vi "command_mapping.vi"(0 "Controls[]":refnum<vi>[](array[refnum]), 2 "cmd in":string, 3 "connection information":path) -> (8 "address out":i16, 9 "value out":T1)   [LabVIEW 2015]
uses:
  Control 1.ctl
  <vilib>/addons/database/Connection.llb/DB Tools Open Connec (Path).vi
  <vilib>/Utility/Data Type/NI_Data Type.lvlib
  <vilib>/addons/database/NI_Database_API.lvlib
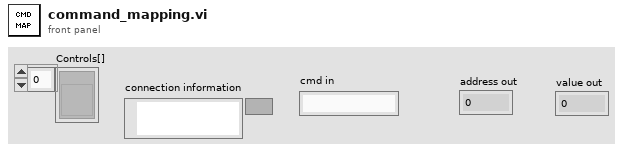
[diagram p1: front panel]
types:
  T1 = typedef "Control 1.ctl" = dbl
  T2 = typedef "NI_Data Type.lvlib/Data Type.ctl" = enum8{"Invalid Type", "Void", "I8", "I16", "I32", "I64", "U8", "U16", "U32", "U64", "Single Float", "Double Float", "Extended Float", "Single Complex", "Double Complex", "Extended Complex", "Enum U8", "Enum U16", "Enum U32", "Enum U64", "Single Float With Unit", "Double Float With Unit", "Extended Float With Unit", "Single Complex with Unit", "Double Complex with Unit", "Extended Complex with Unit", "Boolean", "String", "Path", "Picture", "Tag", "Array", "Cluster", "Variant", "LV Variant", "Waveform", "Timestamp", "Digital Waveform", "Digital Data", "ExpressData", "Refnum", "External Data", "VI", "Poly VI", "LabVIEW Class Instance", "Fixed Point"}
  T3 = typedef "NI_Database_API.lvlib/Conn ObjectReference.ctl" = refnum<k1>
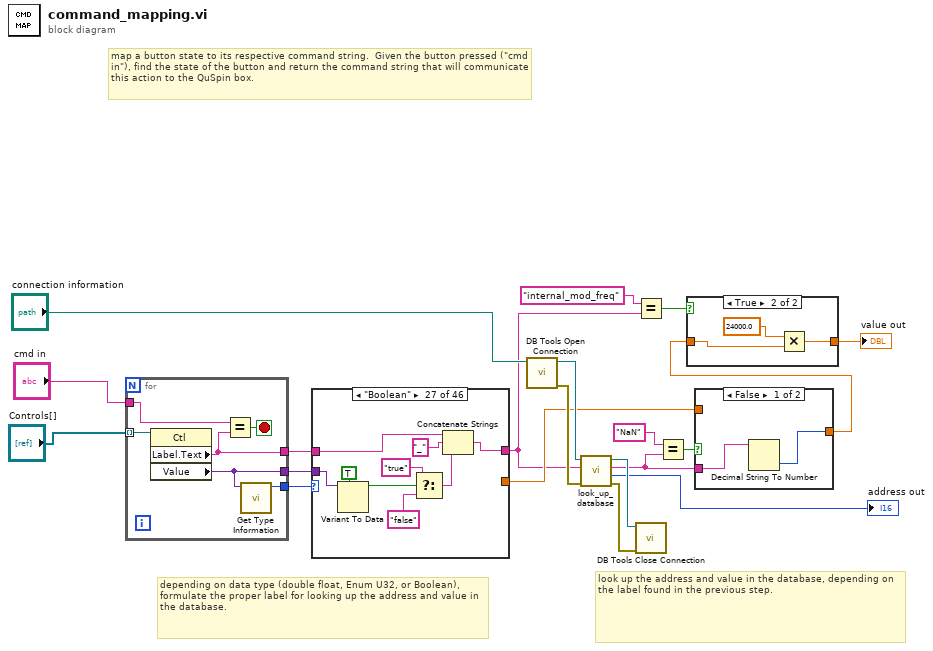
[diagram p0: block diagram]
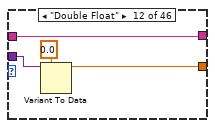
[diagram p15: hidden frame]
diagram:
  # "look up the address and value in the database, depending on the label found in the previous step."
  # "depending on data type (double float, Enum U32, or Boolean), formulate the proper label for looking up the address and value in the database."
  # "map a button state to its respective command string.  Given the button pressed (\"cmd in\"), find the state of the button and return the command string that will communicate this action to the QuSpin box."
  n1 = for {
    tunnel: "Controls[]" -> [w26] mode=indexing
    tunnel: "cmd in" -> [w25]
    tunnel: [w23] -> w18
    tunnel: [w22] -> w17
    tunnel: [w21] -> w16
    stop <- w24 stop-if-true
    n2 = property class="Ctl"(reference=w26) -> ("Label.Text"=w22:string, "Value"=w21:variant)  [unwired: 1 in, 2 out]
    n3 = Equal?(x=w25, y=w22) -> (x = y?=w24:bool)
    n4 = call <vilib>:"Get Type Information.vi"("Variant"=w21) -> ("Type"=w23:T2)  [unwired: 6 in, 4 out]
  }
  n5 = case shown="\"Boolean\"" w18 {
    tunnel: w17 -> [_ _ _ _ _ _ _ _ _ _ _ w28 _ _ _ _ _ _ w38 _ _ _ _ _ _ _ w45 _ _ _ _ _ _ _ _ _ _ _ _ _ _ _ _ _ _ _]
    tunnel: w16 -> [_ _ _ _ _ _ _ _ _ _ _ w30 _ _ _ _ _ _ w35 _ _ _ _ _ _ _ w47 _ _ _ _ _ _ _ _ _ _ _ _ _ _ _ _ _ _ _]
    tunnel: [_ _ _ _ _ _ _ _ _ _ _ w28 _ _ _ _ _ _ w31 _ _ _ _ _ _ _ w39 _ _ _ _ _ _ _ _ _ _ _ _ _ _ _ _ _ _ _] -> w4
    tunnel: [_ _ _ _ _ _ _ _ _ _ _ w29 _ _ _ _ _ _ _ _ _ _ _ _ _ _ _ _ _ _ _ _ _ _ _ _ _ _ _ _ _ _ _ _ _ _] -> w8
    frame "Invalid Type", Default {
    }
    frame "Void" {
    }
    frame "I8" {
    }
    frame "I16" {
    }
    frame "I32" {
    }
    frame "I64" {
    }
    frame "U8" {
    }
    frame "U16" {
    }
    frame "U32" {
    }
    frame "U64" {
    }
    frame "Single Float" {
    }
    frame "Double Float" {
      n6 = Variant To Data(type=0.0, Variant=w30) -> (data=w29:dbl)  [unwired: 1 in, 1 out]
    }
    frame "Extended Float" {
    }
    frame "Single Complex" {
    }
    frame "Double Complex" {
    }
    frame "Extended Complex" {
    }
    frame "Enum U8" {
    }
    frame "Enum U16" {
    }
    frame "Enum U32" {
      n7 = Variant To Data(type=0, Variant=w35) -> (data=w33:i32)  [unwired: 1 in, 1 out]
      n8 = call <vilib>:"Get Numeric Information.vi"("Variant"=w35) -> ("Enum Names"=w34:string[])  [unwired: 7 in, 3 out]
      n9 = Index Array(array=w34, index=w33) -> (element=w32:string)
      n10 = Concatenate Strings(w38, "_" ("string"), w32) -> (w31:string)
    }
    frame "Enum U64" {
    }
    frame "Single Float With Unit" {
    }
    frame "Double Float With Unit" {
    }
    frame "Extended Float With Unit" {
    }
    frame "Single Complex with Unit" {
    }
    frame "Double Complex with Unit" {
    }
    frame "Extended Complex with Unit" {
    }
    frame "Boolean" {
      n11 = Variant To Data(type=TRUE, Variant=w47) -> (data=w43:bool)  [unwired: 1 in, 1 out]
      n12 = Select(t="true", s=w43, f="false") -> (s? t:f=w42:string)
      n13 = Concatenate Strings(w45, "_" ("string"), w42) -> (w39:string)
    }
    frame "String" {
    }
    frame "Path" {
    }
    frame "Picture" {
    }
    frame "Tag" {
    }
    frame "Array" {
    }
    frame "Cluster" {
    }
    frame "Variant" {
    }
    frame "LV Variant" {
    }
    frame "Waveform" {
    }
    frame "Timestamp" {
    }
    frame "Digital Waveform" {
    }
    frame "Digital Data" {
    }
    frame "ExpressData" {
    }
    frame "Refnum" {
    }
    frame "External Data" {
    }
    frame "VI" {
    }
    frame "Poly VI" {
    }
    frame "LabVIEW Class Instance" {
    }
    frame "Fixed Point" {
    }
  }
  n14 = call-poly <vilib>:"DB Tools Open Connection.vi"("connection information"="connection information") -> ("error out"=w14:errorcluster, "connection reference"=w15:T3)  [unwired: 7 in]
  n15 = call "look_up_database.vi"("error in (no error)"=w14, "Label.Text"=w4, "Refnum in"=w15) -> ("error out"=w11:errorcluster, "Numeric"=→"address out":i32, "String"=w6:string, "Refnum out"=w12:T3)  [unwired: 5 in]
  n16 = Equal?(x="internal_mod_freq", y=w4) -> (x = y?=w3:bool)
  n17 = call <vilib>:"DB Tools Close Connection.vi"("error in (no error)"=w11, "connection reference"=w12) -> ()  [unwired: 5 in, 1 out]
  n18 = Equal?(x="NaN", y=w6) -> (x = y?=w9:bool)
  n19 = case shown="False" w9 {
    tunnel: w8 -> [_ w50]
    tunnel: [w48 w50] -> w2
    tunnel: w6 -> [w49 _]
    frame False {
      n20 = Decimal String To Number(string=w49) -> (number=w48:i32)  [unwired: 2 in, 1 out]
    }
    frame True {
    }
  }
  n21 = case shown="True" w3 {
    tunnel: w2 -> [w51 w54]
    tunnel: [w51 w53] -> w1
    frame False {
    }
    frame True {
      n22 = Multiply(x=24000.0, y=w54) -> (x*y=w53:dbl)
    }
  }
  "value out" <- w1
